vi "moveTo.vi"(2 "移动到位置":dbl, 3 "步进电机控制器串口":refnum<visa-resource-name>) -> (0 "字符串":string, 1 "VISA资源名称":refnum<visa-resource-name>)   [LabVIEW 2018]
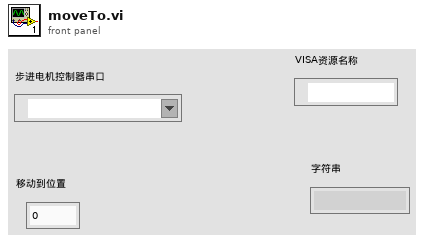
[diagram p1: front panel]
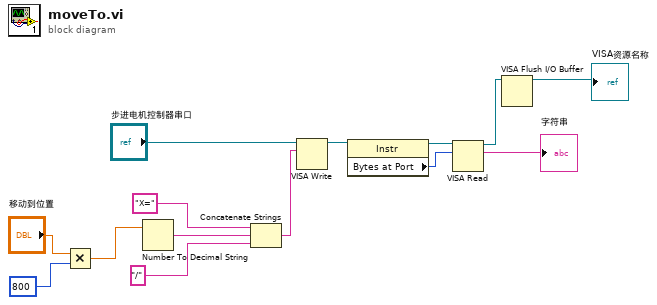
[diagram p0: block diagram]
diagram:
  n1 = Multiply(x="移动到位置", y=800) -> (x*y=w8:dbl)
  n2 = Number To Decimal String(number=w8) -> (decimal integer string=w12:string)  [unwired: 1 in]
  n3 = Concatenate Strings("X=", w12, "/") -> (w11:string)
  n4 = VISA Write(VISA resource name="步进电机控制器串口", write buffer=w11) -> (VISA resource name out=w7:refnum<visa-resource-name>)  [unwired: 1 in, 2 out]
  n5 = property class="Instr"(reference=w7) -> (reference out=w6:refnum<visa-resource-name>, "Bytes at Port"=w5:u32)  [unwired: 1 in, 1 out]
  n6 = VISA Read(VISA resource name=w6, byte count=w5) -> (VISA resource name out=w2:refnum<visa-resource-name>, read buffer=→"字符串":string)  [unwired: 1 in, 2 out]
  n7 = VISA Flush I/O Buffer(VISA resource name=w2) -> (VISA resource name out=→"VISA资源名称":refnum<visa-resource-name>)  [unwired: 2 in, 1 out]
